vi "ImageProcessing_Binarization.vi"(11 "Path":path) -> (3 "Input Image":picture)   [LabVIEW 2020]
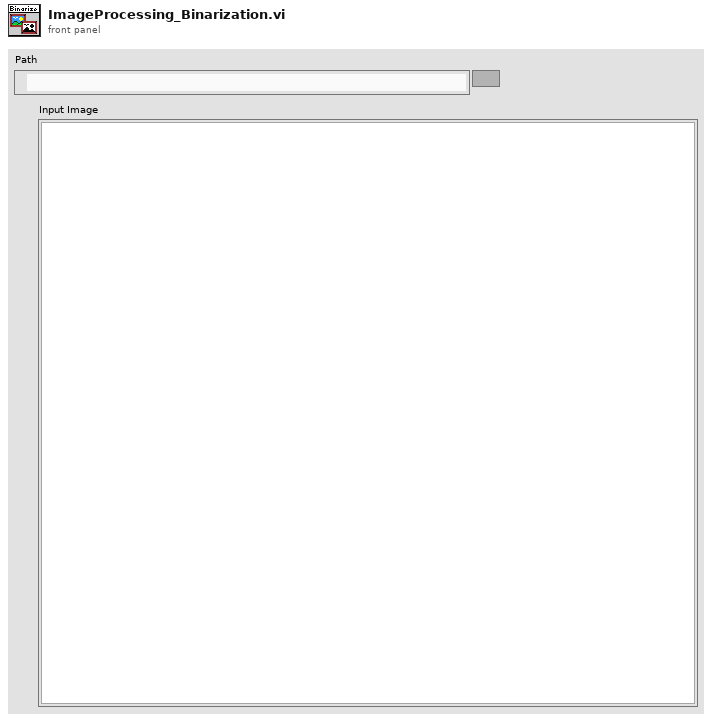
[diagram p1: front panel]
types:
  T1 = typedef "imagedata.ctl" = cluster{"image type":i32, "image depth":i32, "image":u8[], "mask":u8[], "colors":u32[], "Rectangle":cluster{"left":i16, "top":i16, "right":i16, "bottom":i16}}
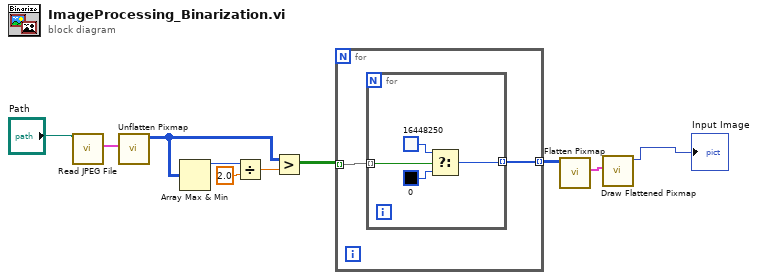
[diagram p0: block diagram]
diagram:
  n1 = call <vilib>:"Read JPEG File.vi"("path to JPEG file"="Path") -> ("image data"=w8:T1)  [unwired: 8 in, 2 out]
  n2 = call <vilib>:"Unflatten Pixmap.vi"("image data"=w8) -> ("24-bit pixmap"=w7:u32[][])  [unwired: 4 in, 6 out]
  n3 = Array Max & Min(array=w7) -> (max value=w4:u32)  [unwired: 3 out]
  n4 = Divide(x=w4, y=2.0) -> (x/y=w5:dbl)
  n5 = Greater?(x=w7, y=w5) -> (0:w6:bool[][])
  n6 = for {
    tunnel: w6 -> [w12] mode=indexing
    tunnel: [w11] -> w2 mode=indexing
    n7 = for {
      tunnel: w12 -> [w16] mode=indexing
      tunnel: [w13] -> w11 mode=indexing
      n8 = Select(t=u32 16448250, s=w16, f=u32 0) -> (s? t:f=w13:u32)
    }
  }
  n9 = call <vilib>:"Flatten Pixmap.vi"("24-bit pixmap"=w2) -> ("image data"=w1:T1)  [unwired: 10 in]
  n10 = call <vilib>:"Draw Flattened Pixmap.vi"("image data"=w1) -> ("new picture"=→"Input Image":picture)  [unwired: 8 in]
